vi "Initialize Channel Array.vi"(8 "error in":errorcluster, 11 "Function Generator in":refnum<class "Function Generator.lvclass">) -> (0 "error out":errorcluster, 3 "Function Generator out":refnum<class "Function Generator.lvclass">)   [LabVIEW 2018, in "Function Generator.lvlib" / "Function Generator.lvclass"]
uses:
  Function Generator.lvclass
  Custom Controls/Channel Settings.ctl
  Custom Controls/Waveform Type.ctl
  Function Generator.lvclass/Function Generator.ctl
  builds/Configuration.lvlibp/Configuration.lvclass
  Function Generator.lvlib
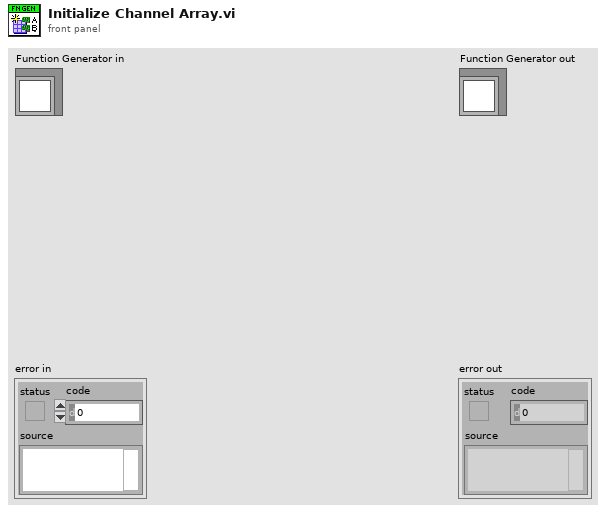
[diagram p1: front panel]
types:
  T1 = typedef "Function Generator.lvlib/Channel Settings.ctl" = cluster{"Waveform Type":T2, "Amplitude Pk-Pk(V)":dbl, "Duty Cycle (%)":dbl, "Frequency (Hz)":dbl, "DC offset":dbl, "Output":bool}
  T2 = typedef "Function Generator.lvlib/Waveform Type.ctl" = enum16{"Sine", "Square", "Triangle", "Sawtooth", "DC"}
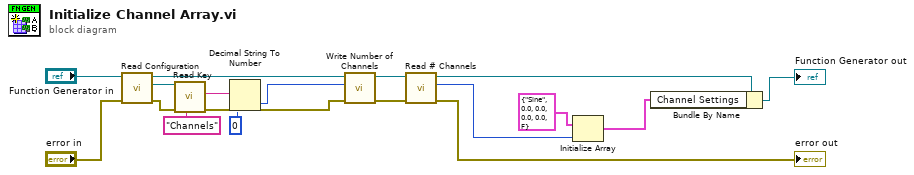
[diagram p0: block diagram]
diagram:
  n1 = call "Read Configuration.vi"("error in (no error)"="error in", "Function Generator in"="Function Generator in") -> ("error out"=w7:errorcluster, "Configuration"=w8:refnum<class "Configuration.lvclass">, "Function Generator out"=w5:refnum<class "Function Generator.lvclass">)  [unwired: 7 in]
  n2 = call "Read Key.vi"("Key:"="Channels", "error in"=w7, "Configuration in"=w8) -> ("error out"=w4:errorcluster, "Value"=w3:string)  [unwired: 6 in, 1 out]
  n3 = Decimal String To Number(string=w3, default (0L)=u8 0) -> (number=w2:u8)  [unwired: 1 in, 1 out]
  n4 = call-dynamic "Write Number of Channels.vi"("error in (no error)"=w4, "# Channels"=w2, "Function Generator in"=w5) -> ("error out"=w18:errorcluster, "Function Generator out"=w17:refnum<class "Function Generator.lvclass">)  [unwired: 7 in]
  n5 = call "Read # Channels.vi"("error in (no error)"=w18, "Function Generator in"=w17) -> ("error out"=→"error out":errorcluster, "# Channels"=w16:u8, "Function Generator out"=w15:refnum<class "Function Generator.lvclass">)  [unwired: 7 in]
  n6 = Initialize Array(T1 {"Waveform Type"=enum."Sine", "Amplitude Pk-Pk(V)"=0.0, "Duty Cycle (%)"=0.0, "Frequency (Hz)"=0.0, "DC offset"=0.0, "Output"=FALSE} ("Channel Settings"), w16) -> (w14:T1[])
  n7 = Bundle By Name(cluster=w15, "Channel Settings"=w14) -> (→"Function Generator out":refnum<class "Function Generator.lvclass">)
